vi "F2.vi"(8 "error in (no error)":errorcluster, 9 "data":u8[](array[numeric]), 10 "function":u8, 11 "device data model in":refnum<class "Standard Data Model.lvclass">) -> (0 "error out":errorcluster, 1 "data return":u8[](array[numeric]), 2 "function return":u8, 3 "device data model out":refnum<class "Standard Data Model.lvclass">)   [LabVIEW 2017, in "SubVIs.lvlib" / "Standard Data Model.lvclass"]
doc: "Executes function code 2"
uses:
  <vilib>/Modbus/subvis/Data and Functions/Standard Data Model/Standard Data Model.lvclass
  <vilib>/Modbus/subvis/SubVIs.lvlib
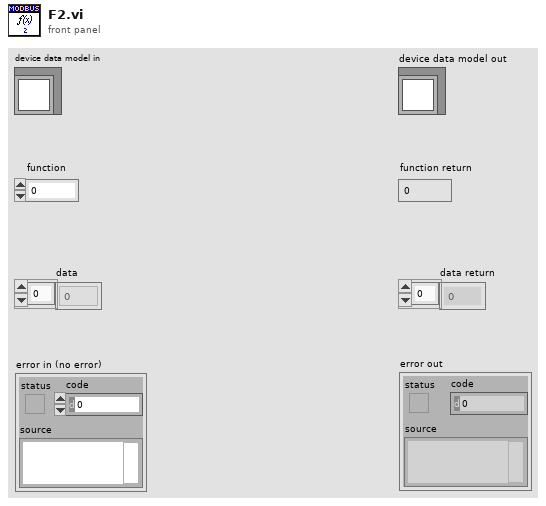
[diagram p1: front panel]
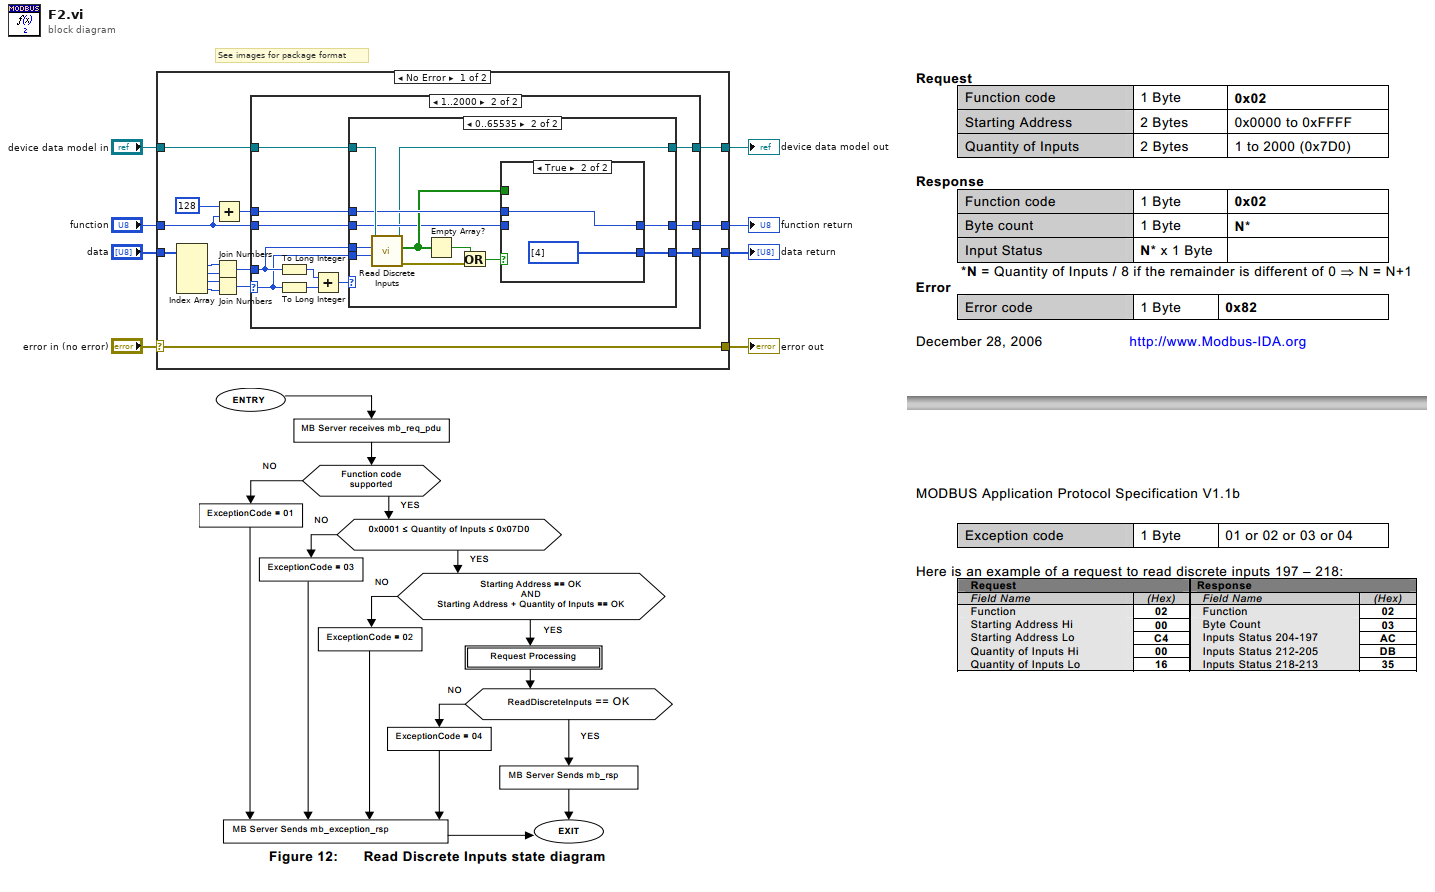
[diagram p0: block diagram]
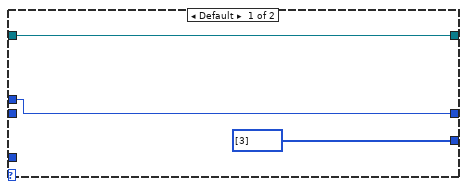
[diagram p2: hidden frame]
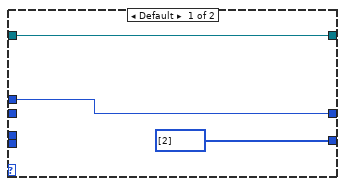
[diagram p3: hidden frame]
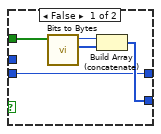
[diagram p4: hidden frame]
diagram:
  # "See images for package format"
  n1 = case shown="No Error" "error in (no error)" {
    selector: "error in (no error)" -> [w23 w63]
    tunnel: [w23 w63] -> w7
    tunnel: [w16 w62] -> w5
    tunnel: "device data model in" -> [w15 w62]
    tunnel: "function" -> [w12 w61]
    tunnel: "data" -> [w18 w60]
    tunnel: [w11 w61] -> w2
    tunnel: [w10 w60] -> w1
    frame No Error {
      n2 = Index Array(array=w18) -> (element #1=w21:u8, element #2=w22:u8, element #3=w20:u8, element #4=w19:u8)  [unwired: 4 in]
      n3 = Join Numbers(hi=w21, lo=w22) -> ((hi.lo)=w9:u16)
      n4 = Join Numbers(hi=w20, lo=w19) -> ((hi.lo)=w17:u16)
      n5 = Add(x=u8 128, y=w12) -> (x+y=w13:u8)
      n6 = case shown="1..2000" w17 {
        selector: w17 -> [_ w33]
        tunnel: [w26 w32] -> w16
        tunnel: w15 -> [w26 w31]
        tunnel: w13 -> [w25 w30]
        tunnel: w12 -> [_ w28]
        tunnel: [w25 w29] -> w11
        tunnel: [u8[] [3] ("Data Return") w27] -> w10
        tunnel: w9 -> [_ w34]
        frame Default {
        }
        frame 1..2000 {
          n7 = To Long Integer(number=w34) -> (32bit integer=w37:i32)
          n8 = To Long Integer(number=w33) -> (32bit integer=w36:i32)
          n9 = Add(x=w37, y=w36) -> (x+y=w35:i32)
          n10 = case shown="0..65535" w35 {
            tunnel: w34 -> [_ w50]
            tunnel: w33 -> [_ w51]
            tunnel: [w40 w41] -> w32
            tunnel: w31 -> [w40 w52]
            tunnel: w30 -> [w39 w47]
            tunnel: [w39 w48] -> w29
            tunnel: w28 -> [_ w44]
            tunnel: [u8[] [2] ("Data Return") w46] -> w27
            frame Default {
            }
            frame 0..65535 {
              n11 = call-dynamic "Read Discrete Inputs.vi"("number of inputs"=w51, "starting address"=w50, "device data model in"=w52) -> ("error out"=w42:errorcluster, "data"=w45:bool[], "device data model out"=w41:refnum<class "Standard Data Model.lvclass">)  [unwired: 6 in]
              n12 = Empty Array?(array=w45) -> (empty?=w43:bool)
              n13 = Or(x=w43, y=w42) -> (x .or. y?=w49:bool)
              n14 = case shown="True" w49 {
                tunnel: [w53 w59] -> w48
                tunnel: w47 -> [_ w59]
                tunnel: [w55 u8[] [4]] -> w46
                tunnel: w45 -> [w54 _]
                tunnel: w44 -> [w53 _]
                frame False {
                  n15 = call <vilib>:"Bits to Bytes.vi"("bits"=w54) -> ("bytes"=w56:u8[], "count"=w57:u8)  [unwired: 9 in]
                  n16 = Build Array (concatenate)(w57, w56) -> (w55:u8[])
                }
                frame True {
                }
              }
            }
          }
        }
      }
    }
    frame Error {
    }
  }
  "error out" <- w7
  "device data model out" <- w5
  "data return" <- w1
  "function return" <- w2
